vi "Write.vi"(8 "error in (no error)":errorcluster, 9 "Variant":variant, 10 "String":string, 11 "VISA in":refnum<class "VISA.lvclass">) -> (0 "error out":errorcluster, 3 "VISA out":refnum<class "VISA.lvclass">)   [LabVIEW 2023, in "Protocols.lvlib" / "VISA.lvclass"]
uses:
  VISA.lvclass
  Protocol Parent/Protocol Parent.lvclass
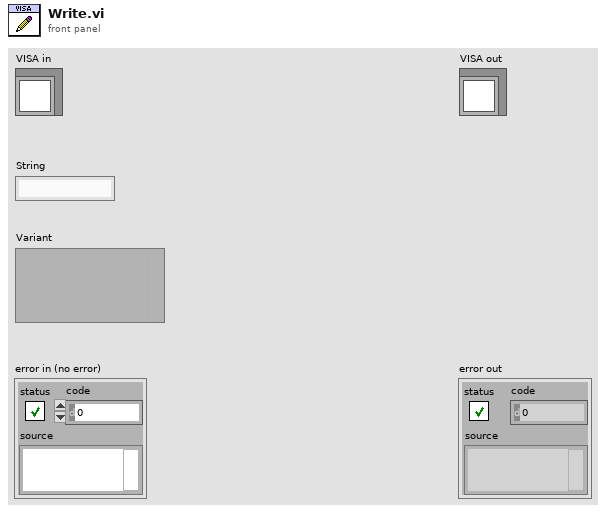
[diagram p1: front panel]
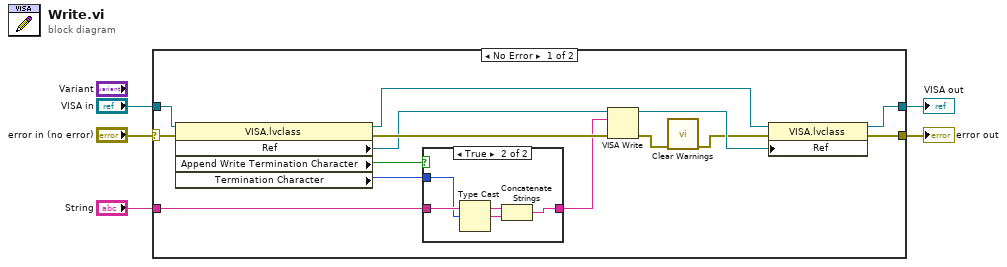
[diagram p0: block diagram]
diagram:
  n1 = case shown="No Error" "error in (no error)" {
    selector: "error in (no error)" -> [w12 w26]
    tunnel: "VISA in" -> [w19 w25]
    tunnel: "String" -> [w10 _]
    tunnel: [w15 w26] -> w2
    tunnel: [w13 w25] -> w1
    frame No Error {
      n2 = property class="VISA.lvclass"(reference=w19, error in=w12) -> (reference out=w14:refnum<class "VISA.lvclass">, error out=w18:errorcluster, "Ref"=w17:refnum<visa-resource-name>, "Append Write Termination Character"=w11:bool, "Termination Character"=w8:u8)
      n3 = case shown="True" w11 {
        tunnel: w10 -> [w20 w24]
        tunnel: [w20 w23] -> w9
        tunnel: w8 -> [_ w22]
        frame False {
        }
        frame True {
          n4 = Type Cast(x=w22) -> (*(type *) &x=w21:string)  [unwired: 1 in]
          n5 = Concatenate Strings(w24, w21) -> (w23:string)
        }
      }
      n6 = VISA Write(VISA resource name=w17, write buffer=w9, error in (no error)=w18) -> (VISA resource name out=w16:refnum<visa-resource-name>, error out=w7:errorcluster)  [unwired: 1 out]
      n7 = call "Clear Warnings.vi"("error in (no error)"=w7) -> ("error out"=w6:errorcluster)  [unwired: 10 in]
      n8 = property class="VISA.lvclass"(reference=w14, error in=w6, "Ref"=w16) -> (reference out=w13:refnum<class "VISA.lvclass">, error out=w15:errorcluster)
    }
    frame Error {
    }
  }
  "error out" <- w2
  "VISA out" <- w1
